vi "Calculate 8h Avg.vi"(8 "error in":errorcluster, 11 "Values in":dbl[][][](array[numeric])) -> (0 "error out":errorcluster, 1 "8h avg":dbl[][](array[numeric]), 3 "Values out":dbl[][][](array[numeric]))   [LabVIEW 2017, in "Akwizycja.lvlib"]
uses:
  Akwizycja.lvlib
panel:
  out "cluster":cluster{"[0]":i32, "[1]":i32, "[2]":i32}
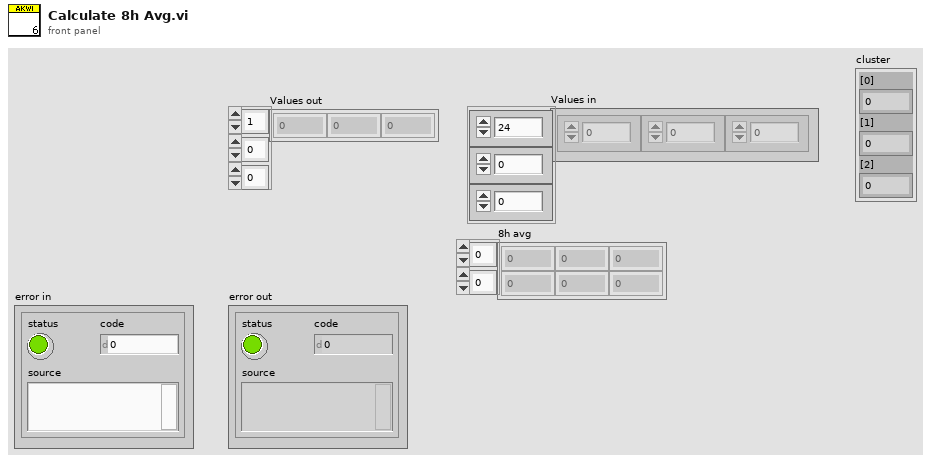
[diagram p1: front panel]
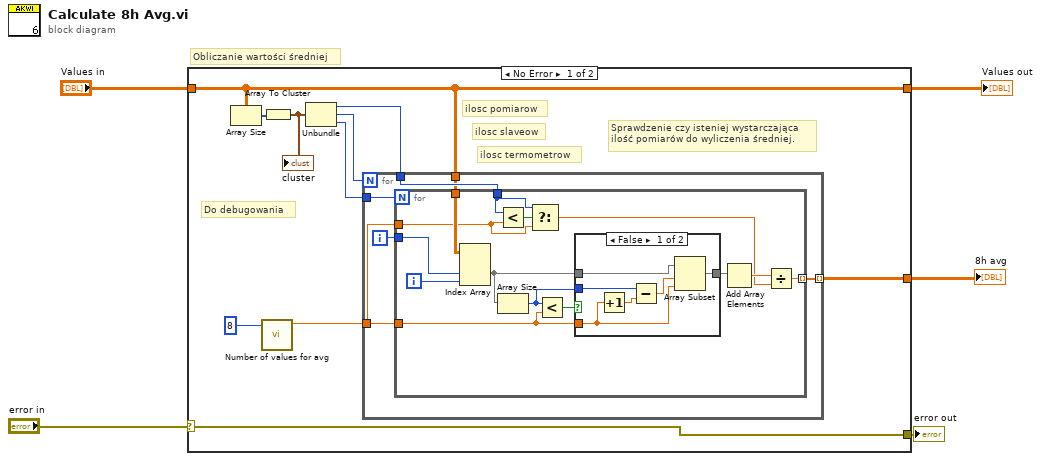
[diagram p0: block diagram]
diagram:
  # "Obliczanie wartości średniej"
  n1 = case shown="No Error" "error in" {
    selector: "error in" -> [w15 w44]
    tunnel: [w15 w44] -> w4
    tunnel: "Values in" -> [w9 w43]
    tunnel: [w9 w43] -> w2
    tunnel: [w8 _] -> w1
    frame No Error {
      # "Do debugowania"
      # "Sprawdzenie czy isteniej wystarczająca \nilość pomiarów do wyliczenia średniej."
      # "Sprawdzenie czy isteniej wystarczająca \nilość pomiarów do wyliczenia średniej."
      # "ilosc termometrow"
      # "ilosc slaveow"
      # "ilosc pomiarow"
      n2 = Array Size(array=w9) -> (size(s)=w14:i32[])
      n3 = call "Number of values for avg.vi"("Avg period (h)"=8 ("Number of values for avg")) -> ("Number of values for avg"=w7:dbl)  [unwired: 9 in, 1 out]
      n4 = Array To Cluster(array=w14) -> (cluster=w13:cluster{"[0]":i32, "[1]":i32, "[2]":i32})
      "cluster" <- w13
      n5 = Unbundle(w13) -> ("[0]"=w10:i32, "[1]"=w12:i32, "[2]"=w11:i32)
      n6 = for {
        N: w12 -> [_]
        tunnel: w11 -> [w21]
        tunnel: w10 -> [w20]
        tunnel: w9 -> [w19]
        tunnel: [w17] -> w8 mode=indexing
        tunnel: w7 -> [w16]
        i -> [w18]
        n7 = for {
          N: w21 -> [_]
          tunnel: w20 -> [w33]
          tunnel: w19 -> [w34]
          tunnel: w18 -> [w32]
          tunnel: [w28] -> w17 mode=indexing
          tunnel: w16 -> [w23]
          tunnel: w16 -> [w22]
          i -> [w31]
          n8 = Index Array(array=w34, index (dim 1)=w32, index (dim 2)=w31) -> (element=w26:dbl[])  [unwired: 1 in]
          n9 = Less?(x=w33, y=w22) -> (x < y?=w35:bool)
          n10 = Array Size(array=w26) -> (size(s)=w24:i32)
          n11 = Select(t=w33, s=w35, f=w22) -> (s? t:f=w29:dbl)
          n12 = Less?(x=w24, y=w23) -> (x < y?=w27:bool)
          n13 = case shown="False" w27 {
            tunnel: w26 -> [w40 w42]
            tunnel: [w41 w42] -> w25
            tunnel: w24 -> [w39 _]
            tunnel: w23 -> [w36 _]
            frame False {
              n14 = Increment(x=w36) -> (x+1=w37:dbl)
              n15 = Subtract(x=w39, y=w37) -> (x-y=w38:dbl)
              n16 = Array Subset(array=w40, index=w38, length=w36) -> (w41:dbl[])
            }
            frame True {
            }
          }
          n17 = Add Array Elements(numeric array=w25) -> (sum=w30:dbl)
          n18 = Divide(x=w30, y=w29) -> (x/y=w28:dbl)
        }
      }
    }
    frame Error {
    }
  }
  "error out" <- w4
  "Values out" <- w2
  "8h avg" <- w1
